vi "pco.camera_FloatingMean_Example_IMAQ.vi"() -> ()   [LabVIEW 2019]
uses:
  pco.camera/Camera.lvclass
  <vilib>/vision/NI_Vision_Development_Module.lvlib
panel:
  out "nominatorU64":u64 format="%x"
  out "denominatorU64":u64 format="%x"
  out "currentImage":T1(plugin-control)
  out "nominatorU32":u64 format="%x"
  out "denominatorU32":u64 format="%x"
  in  "averageCount":u8=10 caption="Average Count" min=2
  out "Image":T1(plugin-control)
  in  "data_format":T2(ring)=enum."Mono16"
  out "Recorded Images":u32
  in  "Quit":bool
  in  "roiY1":u64=2048 min=2 max=20000 step=1
  in  "roiX1":u64=2048 min=2 max=20000 step=1
  in  "roiY0":u64=1 min=1 max=1039 step=1
  in  "roiX0":u64=1 min=1 max=1391 step=1
  out "Image Height":u64
  out "Image Width":u64
  in  "dwImgCount":u32=10 caption="Fifo Buffer Size" max=4023
  out "Error":errorcluster {"code" format="%x"}
  # "This example shows how to compute and show a floating mean live image.\nHere the camera class is operated in fifo mode to always get next image in buffer.\nThe Average Count defines the number of images that will be averaged.\nAveraging is done by fetiching one image and using average image from previous iteration\n(avg_n = (1-1/avg_count)*avg_(n-1) + (1/avg_count)*image_n)\n\nIt is a good starting point for writing own applications.\nBut it will not be fail save, i.e. doesnt react on errors, just handles them forward to the end\n\nUsage:\nSelect your required fifo buffer size and image format and start the program.\nOnce started, the camera class will be initialized and image record will start automatically.\nInside the acquisition loop the program calculates the floating average image shows it.\nThe average count can be changed at any time.\nBy using the ROI parameters you can crop the image to select certain regions\n\nBy clicking Quit Application the record will stop and will force an exit of the camera class"
  # "pco.labview"
  # "Camera Setup"
  # "Recording Control"
  # "Parameters for image readout"
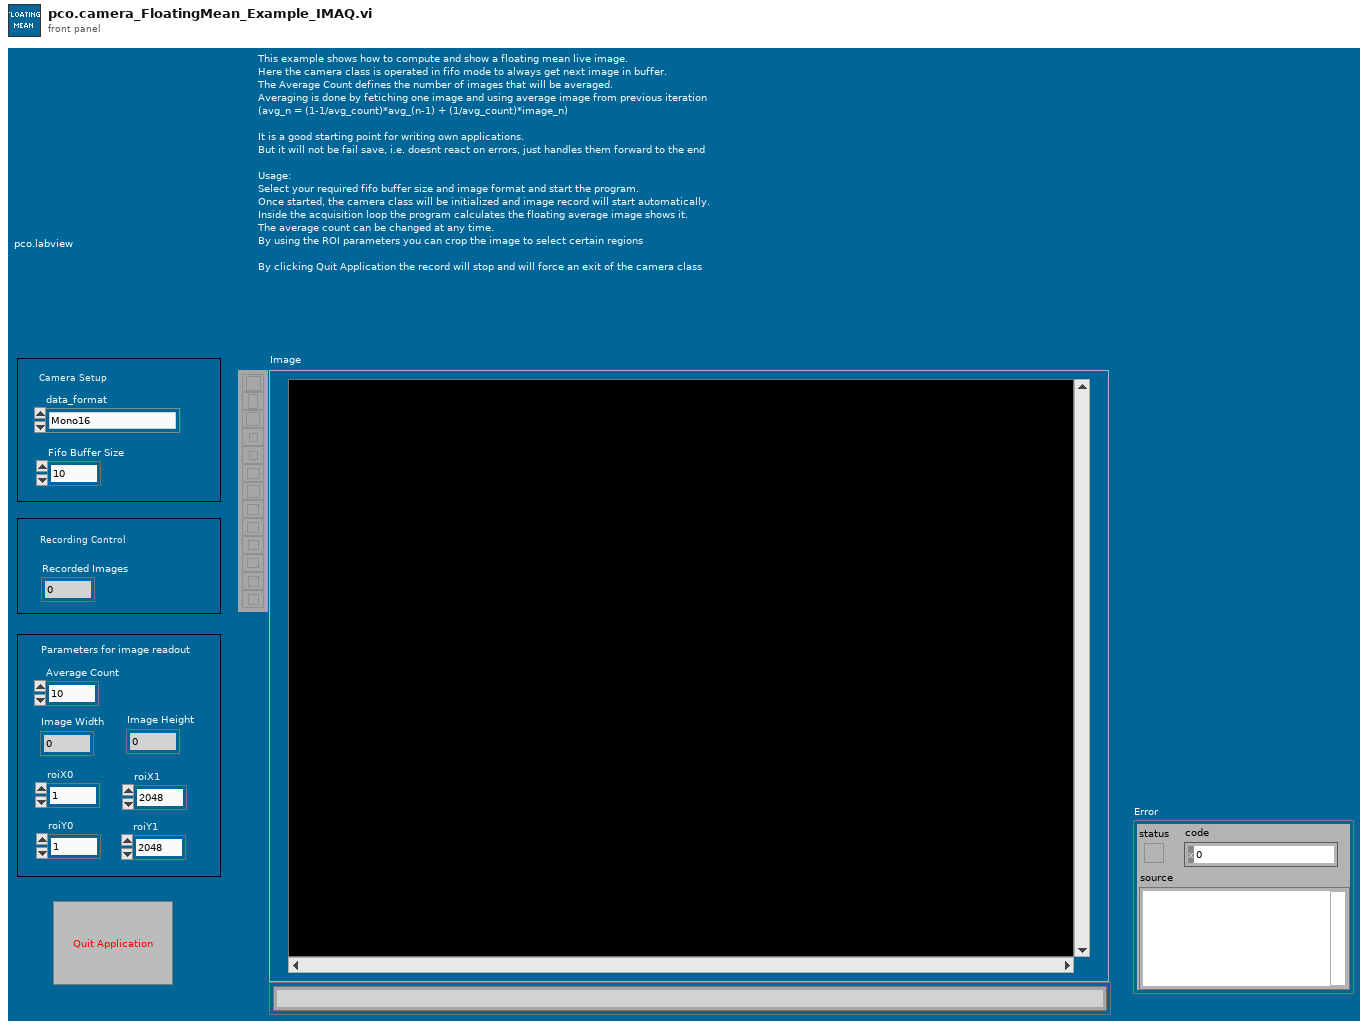
[diagram p1: front panel]
types:
  T1 = typedef "IMAQ Image.ctl" = refnum<image>
  T2 = enum16{"Undefined", "Mono8", "Mono16", "BGRA8", "RGBA8", "BGRA16", "RGBA16", "CompressedMono8"}
  T3 = enum8{"Enabled", "Disabled", "Disabled and Grayed Out"}
  T4 = enum16{"sequence", "sequence non blocking", "ring buffer", "fifo", "sequence_dpcore", "sequence_non_blocking_dpcore", "ring_buffer_dpcore", "fifo_dpcore", "tif", "multitif", "pcoraw", "b16", "dicom", "multidicom"}
  T5 = typedef "Image Type" = u32
  T6 = typedef "Camera.lvclass/binning.ctl" = cluster{"vert":u16, "horz":u16}
  T7 = cluster{"exposure_time_s":dbl, "delay_time_s":dbl, "roi":cluster{"x0":u64, "y0":u64, "x1":u64, "y1":u64}, "timestamp_mode":u16, "pixelrate":u32, "trigger_mode":u16, "acquire_mode":u16, "metadata_mode":u16, "noisefilter_mode":u16, "binning":T6}
  T8 = typedef "Color (U64)" = cluster{"Plane 3 (Blue)":u16, "Plane 2 (Green)":u16, "Plane 1 (Red)":u16, "Plane 4 (alpha)":u16}
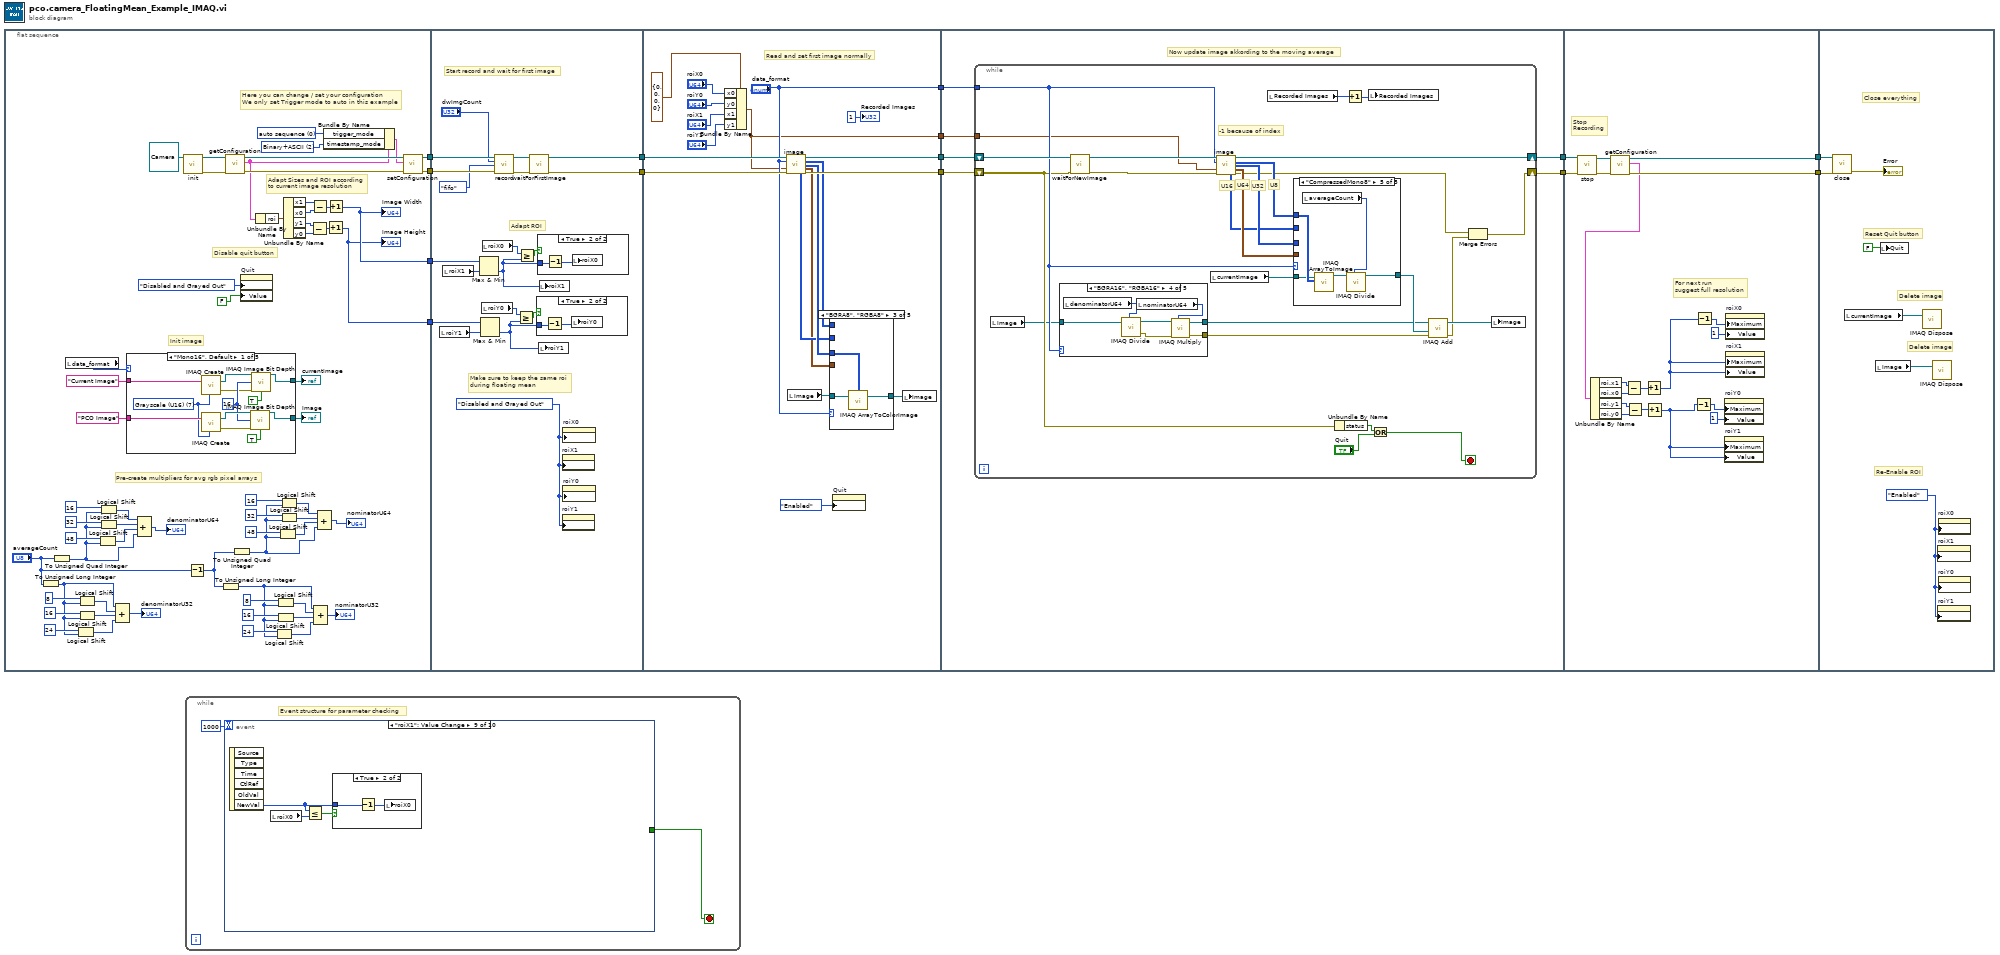
[diagram p0: block diagram]
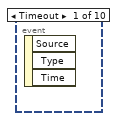
[diagram p2: hidden frame]
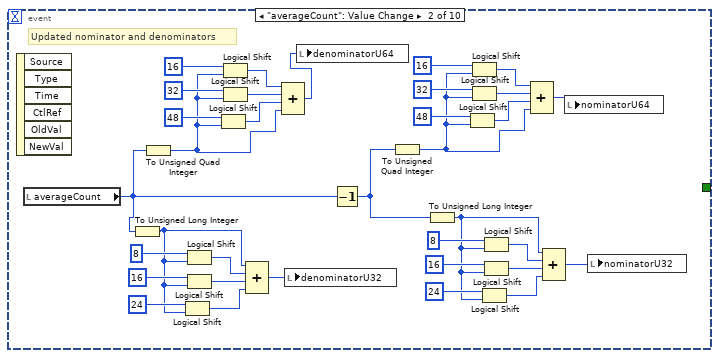
[diagram p3: hidden frame]
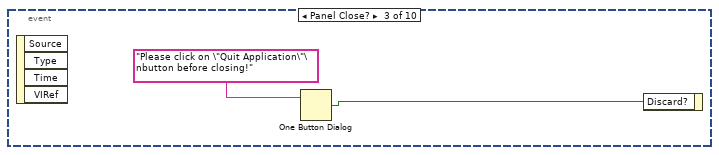
[diagram p4: hidden frame]
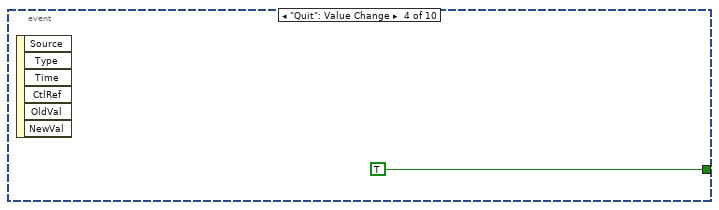
[diagram p5: hidden frame]
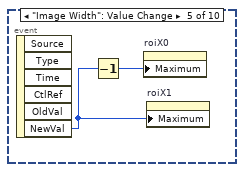
[diagram p6: hidden frame]
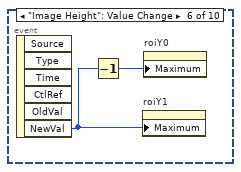
[diagram p7: hidden frame]
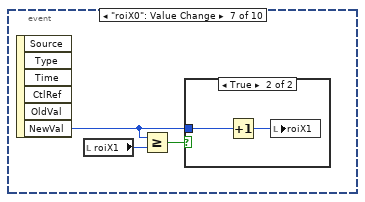
[diagram p8: hidden frame]
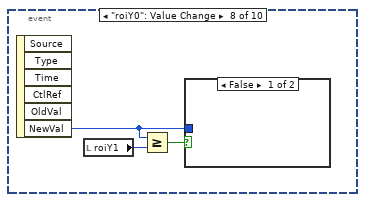
[diagram p10: hidden frame]
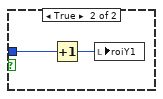
[diagram p11: hidden frame]
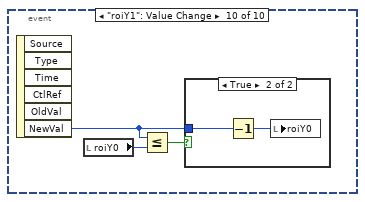
[diagram p13: hidden frame]
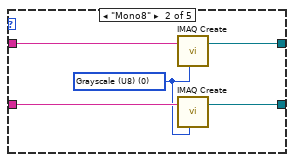
[diagram p15: hidden frame]
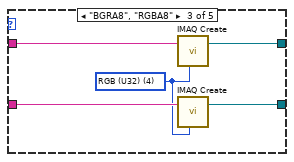
[diagram p16: hidden frame]
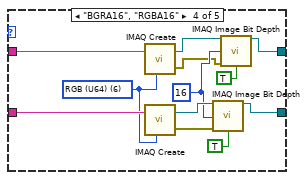
[diagram p17: hidden frame]
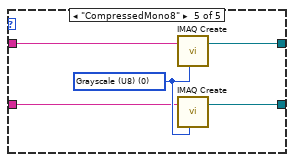
[diagram p18: hidden frame]
diagram:
  n1 = flat-sequence {
    tunnel: [w68] -> w14
    tunnel: [w67] -> w13
    tunnel: [w16] -> w2
    tunnel: [w15] -> w1
    tunnel: w14 -> [w133]
    tunnel: w13 -> [w132]
    tunnel: [w127] -> w12
    tunnel: [w126] -> w11
    tunnel: w2 -> [w123]
    tunnel: w1 -> [w121]
    tunnel: w12 -> [w155]
    tunnel: w11 -> [w154]
    tunnel: [w150] -> w10
    tunnel: [w151] -> w9
    tunnel: ["data_format"] -> w4
    tunnel: [w138] -> w3
    tunnel: w10 -> [w176]
    tunnel: w9 -> [w177]
    tunnel: [w175] -> w8
    tunnel: [w174] -> w6
    tunnel: w4 -> [w173]
    tunnel: w3 -> [w172]
    tunnel: w8 -> [w281]
    tunnel: [w276] -> w7
    tunnel: w6 -> [w280]
    tunnel: [w277] -> w5
    tunnel: w7 -> [w286]
    tunnel: w5 -> [w285]
    frame #0 {
      w58 = u16 2 items=["OFF", "Binary", "Binary+ASCII", "ASCII"] ("TimestampMode")
      w72 = u16 0 items=["auto sequence"=0, "software trigger"=1, "external exposure start & software trigger"=2, "external exposure control"=3, "external synchronized"=4, "fast external exposure control"=5, "external CDS control"=6, "slow external exposure control"=7, "external synchronized HDSDI"=258] ("TriggerMode")
      # "Pre-create multipliers for avg rgb pixel arrays"
      # "Init image"
      # "Adapt Sizes and ROI according\nto current image resolution"
      # "Disable quit button"
      # "Here you can change / set your configuration\nWe only set Trigger mode to auto in this example"
      n2 = To Unsigned Long Integer(number="averageCount") -> (unsigned 32bit integer=w38:u32)
      n3 = To Unsigned Quad Integer(1:"averageCount") -> (0:w18:u64)
      n4 = local read "data_format"() -> (w55:T2)
      n5 = Logical Shift(y=u32 24, x=w38) -> (x << y=w49:u32)
      n6 = Logical Shift(y=u32 8, x=w38) -> (x << y=w47:u32)
      n7 = Logical Shift(y=u32 16, x=w38) -> (x << y=w48:u32)
      n8 = Logical Shift(y=u32 48, x=w18) -> (x << y=w31:u64)
      n9 = Logical Shift(y=u32 16, x=w18) -> (x << y=w29:u64)
      n10 = Logical Shift(y=u32 32, x=w18) -> (x << y=w30:u64)
      n11 = Compound Arithmetic op=ADD(w38, w47, w48, w49) -> (→"denominatorU32":u32)
      n12 = case shown="\"Mono16\", Default" w55 {
        tunnel: "PCO Image" ("Image Name") -> [w87 w90 w95 w109 w112]
        tunnel: [w81 w92 w97 w103 w114] -> w54
        tunnel: [w76 w91 w96 w99 w111] -> w36
        tunnel: "Current Image" ("Image Name") -> [w85 w89 w93 w107 w110]
        frame "Mono16", Default {
          w79 = u32 16 ("Bit Depth (0)")
          w86 = T5 7 items=["Grayscale (U8)", "Grayscale (I16)", "Grayscale (SGL)", "Complex (CSG)", "RGB (U32)", "HSL (U32)", "RGB (U64)", "Grayscale (U16)"] ("Image Type")
          n13 = call "IMAQ Create"("Image Name"=w85, "Image Type"=w86) -> ("New Image"=w78:T1, "error out"=w77:errorcluster)  [unwired: 3 in]
          n14 = call "IMAQ Create"("Image Name"=w87, "Image Type"=w86) -> ("New Image"=w83:T1, "error out"=w82:errorcluster)  [unwired: 3 in]
          n15 = call "IMAQ Image Bit Depth"("Image"=w83, "Bit Depth (0)"=w79, "error in (no error)"=w82, "Get/Set Bit Depth? (Set)"=TRUE) -> ("Image Out"=w81:T1)  [unwired: 9 in, 2 out]
          n16 = call "IMAQ Image Bit Depth"("Image"=w78, "Bit Depth (0)"=w79, "error in (no error)"=w77, "Get/Set Bit Depth? (Set)"=TRUE) -> ("Image Out"=w76:T1)  [unwired: 9 in, 2 out]
        }
        frame "Mono8" {
          w88 = T5 0 items=["Grayscale (U8)", "Grayscale (I16)", "Grayscale (SGL)", "Complex (CSG)", "RGB (U32)", "HSL (U32)", "RGB (U64)", "Grayscale (U16)"] ("Image Type")
          n17 = call "IMAQ Create"("Image Name"=w89, "Image Type"=w88) -> ("New Image"=w91:T1)  [unwired: 3 in, 1 out]
          n18 = call "IMAQ Create"("Image Name"=w90, "Image Type"=w88) -> ("New Image"=w92:T1)  [unwired: 3 in, 1 out]
        }
        frame "BGRA8", "RGBA8" {
          w94 = T5 4 items=["Grayscale (U8)", "Grayscale (I16)", "Grayscale (SGL)", "Complex (CSG)", "RGB (U32)", "HSL (U32)", "RGB (U64)", "Grayscale (U16)"] ("Image Type")
          n19 = call "IMAQ Create"("Image Name"=w93, "Image Type"=w94) -> ("New Image"=w96:T1)  [unwired: 3 in, 1 out]
          n20 = call "IMAQ Create"("Image Name"=w95, "Image Type"=w94) -> ("New Image"=w97:T1)  [unwired: 3 in, 1 out]
        }
        frame "BGRA16", "RGBA16" {
          w101 = u32 16 ("Bit Depth (0)")
          w108 = T5 6 items=["Grayscale (U8)", "Grayscale (I16)", "Grayscale (SGL)", "Complex (CSG)", "RGB (U32)", "HSL (U32)", "RGB (U64)", "Grayscale (U16)"] ("Image Type")
          n21 = call "IMAQ Create"("Image Name"=w107, "Image Type"=w108) -> ("New Image"=w100:T1, "error out"=w98:errorcluster)  [unwired: 3 in]
          n22 = call "IMAQ Create"("Image Name"=w109, "Image Type"=w108) -> ("New Image"=w105:T1, "error out"=w104:errorcluster)  [unwired: 3 in]
          n23 = call "IMAQ Image Bit Depth"("Image"=w105, "Bit Depth (0)"=w101, "error in (no error)"=w104, "Get/Set Bit Depth? (Set)"=TRUE) -> ("Image Out"=w103:T1)  [unwired: 9 in, 2 out]
          n24 = call "IMAQ Image Bit Depth"("Image"=w100, "Bit Depth (0)"=w101, "error in (no error)"=w98, "Get/Set Bit Depth? (Set)"=TRUE) -> ("Image Out"=w99:T1)  [unwired: 9 in, 2 out]
        }
        frame "CompressedMono8" {
          w113 = T5 0 items=["Grayscale (U8)", "Grayscale (I16)", "Grayscale (SGL)", "Complex (CSG)", "RGB (U32)", "HSL (U32)", "RGB (U64)", "Grayscale (U16)"] ("Image Type")
          n25 = call "IMAQ Create"("Image Name"=w110, "Image Type"=w113) -> ("New Image"=w111:T1)  [unwired: 3 in, 1 out]
          n26 = call "IMAQ Create"("Image Name"=w112, "Image Type"=w113) -> ("New Image"=w114:T1)  [unwired: 3 in, 1 out]
        }
      }
      "Image" <- w54
      "currentImage" <- w36
      n27 = Compound Arithmetic op=ADD(w29, w30, w31, w18) -> (→"denominatorU64":u64)
      n28 = call-dynamic "init.vi"("Camera in"=refnum<class "Camera.lvclass"> refnum ("PCOCamera in")) -> ("Camera out"=w74:refnum<class "Camera.lvclass">, "error out"=w73:errorcluster)  [unwired: 8 in]
      n29 = Decrement(x="averageCount") -> (x-1=w19:u8)
      n30 = To Unsigned Long Integer(number=w19) -> (unsigned 32bit integer=w37:u32)
      n31 = call-dynamic "getConfiguration.vi"("error in (no error)"=w73, "Camera in"=w74) -> ("error out"=w70:errorcluster, "configuration"=w66:T7, "Camera out"=w71:refnum<class "Camera.lvclass">)  [unwired: 7 in]
      n32 = To Unsigned Quad Integer(1:w19) -> (0:w17:u64)
      n33 = property on="Quit" class="Bool (strict)"("DisabledEnum"=T3."Disabled and Grayed Out" ("Disabled"), "Value"=FALSE ("Stop")) -> ()  [unwired: 2 in, 2 out]
      n34 = Unbundle By Name(w66) -> ("roi"=w65:cluster{"x0":u64, "y0":u64, "x1":u64, "y1":u64})
      n35 = Logical Shift(y=u32 24, x=w37) -> (x << y=w42:u32)
      n36 = Logical Shift(y=u32 8, x=w37) -> (x << y=w40:u32)
      n37 = Logical Shift(y=u32 16, x=w37) -> (x << y=w41:u32)
      n38 = Logical Shift(y=u32 48, x=w17) -> (x << y=w23:u64)
      n39 = Logical Shift(y=u32 16, x=w17) -> (x << y=w25:u64)
      n40 = Logical Shift(y=u32 32, x=w17) -> (x << y=w24:u64)
      n41 = Unbundle By Name(w65) -> ("x1"=w63:u64, "x0"=w64:u64, "y1"=w61:u64, "y0"=w62:u64)
      n42 = Subtract(x=w61, y=w62) -> (x-y=w59:u64)
      n43 = Subtract(x=w63, y=w64) -> (x-y=w60:u64)
      n44 = Compound Arithmetic op=ADD(w37, w40, w41, w42) -> (→"nominatorU32":u32)
      n45 = Compound Arithmetic op=ADD(w25, w24, w23, w17) -> (→"nominatorU64":u64)
      n46 = Bundle By Name(cluster=w66, "trigger_mode"=w72, "timestamp_mode"=w58) -> (w69:T7)
      n47 = Increment(x=w59) -> (x+1=w15:u64)
      "Image Height" <- w15
      n48 = Increment(x=w60) -> (x+1=w16:u64)
      "Image Width" <- w16
      n49 = call-dynamic "setConfiguration.vi"("error in (no error)"=w70, "configuration"=w69, "Camera in"=w71) -> ("error out"=w67:errorcluster, "Camera out"=w68:refnum<class "Camera.lvclass">)  [unwired: 7 in]
    }
    frame #1 {
      w125 = T3."Disabled and Grayed Out" ("Disabled")
      # "Adapt ROI"
      # "Make sure to keep the same roi\nduring floating mean"
      # "Start record and wait for first image"
      n50 = local read "roiY1"() -> (w122:u64)
      n51 = local read "roiX1"() -> (w124:u64)
      n52 = Max & Min(x=w123, y=w124) -> (min(x,y)=w118:u64)  [unwired: 1 out]
      n53 = Max & Min(x=w121, y=w122) -> (min(x,y)=w115:u64)  [unwired: 1 out]
      n54 = local read "roiY0"() -> (w116:u64)
      n55 = local read "roiX0"() -> (w120:u64)
      n56 = call-dynamic "record.vi"("Camera in"=w133, "num_images"="dwImgCount", "record_mode"=T4."fifo", "error in (no error)"=w132) -> ("Camera out"=w128:refnum<class "Camera.lvclass">, "error out"=w129:errorcluster)  [unwired: 10 in]
      n57 = Greater Or Equal?(x=w116, y=w115) -> (x >= y?=w117:bool)
      n58 = Greater Or Equal?(x=w120, y=w118) -> (x >= y?=w119:bool)
      n59 = call-dynamic "waitForFirstImage.vi"("error in (no error)"=w129, "Camera in"=w128) -> ("error out"=w126:errorcluster, "Camera out"=w127:refnum<class "Camera.lvclass">)  [unwired: 8 in]
      n60 = case shown="True" w117 {
        tunnel: w115 -> [_ w135]
        frame False {
        }
        frame True {
          n61 = Decrement(x=w135) -> (x-1=w134:u64)
          n62 = local write "roiY0"(w134) -> ()
        }
      }
      n63 = case shown="True" w119 {
        tunnel: w118 -> [_ w137]
        frame False {
        }
        frame True {
          n64 = Decrement(x=w137) -> (x-1=w136:u64)
          n65 = local write "roiX0"(w136) -> ()
        }
      }
      n66 = local write "roiY1"(w115) -> ()
      n67 = local write "roiX1"(w118) -> ()
      n68 = property on="roiX1" class="DigNum (strict)"("DisabledEnum"=w125) -> ()  [unwired: 2 in, 2 out]
      n69 = property on="roiY1" class="DigNum (strict)"("DisabledEnum"=w125) -> ()  [unwired: 2 in, 2 out]
      n70 = property on="roiX0" class="DigNum (strict)"("DisabledEnum"=w125) -> ()  [unwired: 2 in, 2 out]
      n71 = property on="roiY0" class="DigNum (strict)"("DisabledEnum"=w125) -> ()  [unwired: 2 in, 2 out]
    }
    frame #2 {
      # "Read and set first image normally"
      n72 = Bundle By Name(cluster=cluster{"x0":u64, "y0":u64, "x1":u64, "y1":u64} {"x0"=0, "y0"=0, "x1"=0, "y1"=0} ("roi"), "x0"="roiX0", "y0"="roiY0", "x1"="roiX1", "y1"="roiY1") -> (w138:cluster{"x0":u64, "y0":u64, "x1":u64, "y1":u64})
      n73 = call-dynamic "image.vi"("Camera in"=w155, "data_format"="data_format", "roi"=w138, "error in (no error)"=w154) -> ("Camera out"=w150:refnum<class "Camera.lvclass">, "image (U8)"=w148:u8[][], "image (U32)"=w147:u32[][], "image (U64)"=w145:T8[][], "raw_image (U16)"=w146:u16[][], "error out"=w151:errorcluster)  [unwired: 4 in, 2 out]
      n74 = local read "Image"() -> (w153:T1)
      n75 = case shown="\"BGRA8\", \"RGBA8\"" "data_format" {
        tunnel: w153 -> [w159 w162 w163 w168 w171]
        tunnel: [w157 w160 w165 w166 w170] -> w144
        tunnel: w145 -> [_ _ _ w167 _]
        tunnel: w147 -> [_ _ w164 _ _]
        tunnel: w148 -> [_ w161 _ _ w169]
        tunnel: w146 -> [w158 _ _ _ _]
        frame "Mono16", Default {
          n76 = call "IMAQ ArrayToImage"("Image Pixels (U16)"=w158, "Image"=w159) -> ("Image Out"=w157:T1)  [unwired: 8 in, 1 out]
        }
        frame "Mono8" {
          n77 = call "IMAQ ArrayToImage"("Image Pixels (U8)"=w161, "Image"=w162) -> ("Image Out"=w160:T1)  [unwired: 8 in, 1 out]
        }
        frame "BGRA8", "RGBA8" {
          n78 = call "IMAQ ArrayToColorImage"("Image Pixels (U32)"=w164, "Image"=w163) -> ("Image Out"=w165:T1)  [unwired: 3 in, 1 out]
        }
        frame "BGRA16", "RGBA16" {
          n79 = call "IMAQ ArrayToColorImage"("Image"=w168, "Image Pixels (U64)"=w167) -> ("Image Out"=w166:T1)  [unwired: 3 in, 1 out]
        }
        frame "CompressedMono8" {
          n80 = call "IMAQ ArrayToImage"("Image Pixels (U8)"=w169, "Image"=w171) -> ("Image Out"=w170:T1)  [unwired: 8 in, 1 out]
        }
      }
      n81 = property on="Quit" class="Bool (strict)"("DisabledEnum"=T3."Enabled" ("Disabled")) -> ()  [unwired: 2 in, 2 out]
      n82 = local write "Image"(w144) -> ()
      "Recorded Images" <- u32 1 ("Recorded Images")
    }
    frame #3 {
      # "Now update image akkording to the moving average"
      n83 = while {
        shift-right: [w202] -> w175
        shift-left: w176 -> [w201]
        shift-right: [w182] -> w174
        shift-left: w177 -> [w188]
        tunnel: w173 -> [w191]
        tunnel: w172 -> [w178]
        stop <- w185 stop-if-true
        # "-1 because of index"
        # "U64"
        # "U32"
        # "U16"
        # "U8"
        n84 = local read "Image"() -> (w181:T1)
        n85 = case shown="\"BGRA16\", \"RGBA16\"" w191 {
          tunnel: w181 -> [w206 w214 w222 w229 w235]
          tunnel: [w205 w212 w219 w228 w233] -> w179
          tunnel: [w203 w210 w217 w226 w231] -> w189
          frame "Mono16", Default {
            n86 = local read "averageCount"() -> (w208:u8)
            n87 = call "IMAQ Divide"("Image Src A"=w206, "Constant"=w208) -> ("Image Dst Out"=w209:T1, "error out"=w204:errorcluster)  [unwired: 5 in]
            n88 = Decrement(x=w208) -> (x-1=w207:u8)
            n89 = call "IMAQ Multiply"("Image Src A"=w209, "Constant"=w207, "error in (no error)"=w204) -> ("Image Dst Out"=w205:T1, "error out"=w203:errorcluster)  [unwired: 4 in]
          }
          frame "Mono8" {
            n90 = local read "averageCount"() -> (w213:u8)
            n91 = call "IMAQ Divide"("Image Src A"=w214, "Constant"=w213) -> ("Image Dst Out"=w216:T1, "error out"=w211:errorcluster)  [unwired: 5 in]
            n92 = Decrement(x=w213) -> (x-1=w215:u8)
            n93 = call "IMAQ Multiply"("Image Src A"=w216, "Constant"=w215, "error in (no error)"=w211) -> ("Image Dst Out"=w212:T1, "error out"=w210:errorcluster)  [unwired: 4 in]
          }
          frame "BGRA8", "RGBA8" {
            n94 = local read "denominatorU32"() -> (w221:u64)
            n95 = call "IMAQ Divide"("Image Src A"=w222, "Constant"=w221) -> ("Image Dst Out"=w223:T1, "error out"=w218:errorcluster)  [unwired: 5 in]
            n96 = local read "nominatorU32"() -> (w220:u64)
            n97 = call "IMAQ Multiply"("Image Src A"=w223, "Constant"=w220, "error in (no error)"=w218) -> ("Image Dst Out"=w219:T1, "error out"=w217:errorcluster)  [unwired: 4 in]
          }
          frame "BGRA16", "RGBA16" {
            n98 = local read "denominatorU64"() -> (w225:u64)
            n99 = call "IMAQ Divide"("Image Src A"=w229, "Constant"=w225) -> ("Image Dst Out"=w230:T1, "error out"=w227:errorcluster)  [unwired: 5 in]
            n100 = local read "nominatorU64"() -> (w224:u64)
            n101 = call "IMAQ Multiply"("Image Src A"=w230, "Constant"=w224, "error in (no error)"=w227) -> ("Image Dst Out"=w228:T1, "error out"=w226:errorcluster)  [unwired: 4 in]
          }
          frame "CompressedMono8" {
            n102 = local read "averageCount"() -> (w234:u8)
            n103 = call "IMAQ Divide"("Image Src A"=w235, "Constant"=w234) -> ("Image Dst Out"=w237:T1, "error out"=w232:errorcluster)  [unwired: 5 in]
            n104 = Decrement(x=w234) -> (x-1=w236:u8)
            n105 = call "IMAQ Multiply"("Image Src A"=w237, "Constant"=w236, "error in (no error)"=w232) -> ("Image Dst Out"=w233:T1, "error out"=w231:errorcluster)  [unwired: 4 in]
          }
        }
        n106 = call-dynamic "waitForNewImage.vi"("error in (no error)"=w188, "Camera in"=w201) -> ("error out"=w197:errorcluster, "Camera out"=w198:refnum<class "Camera.lvclass">)  [unwired: 8 in]
        n107 = local read "currentImage"() -> (w190:T1)
        n108 = call-dynamic "image.vi"("Camera in"=w198, "data_format"=w191, "roi"=w178, "error in (no error)"=w197) -> ("Camera out"=w202:refnum<class "Camera.lvclass">, "image (U8)"=w196:u8[][], "image (U32)"=w194:u32[][], "image (U64)"=w195:T8[][], "raw_image (U16)"=w193:u16[][], "error out"=w183:errorcluster)  [unwired: 4 in, 2 out]
        n109 = local read "Recorded Images"() -> (w200:u32)
        n110 = case shown="\"CompressedMono8\"" w191 {
          tunnel: [w239 w245 w250 w255 w259] -> w180
          tunnel: w195 -> [_ _ _ w257 _]
          tunnel: w194 -> [_ _ w252 _ _]
          tunnel: w196 -> [_ w247 _ _ w262]
          tunnel: w193 -> [w242 _ _ _ _]
          tunnel: w190 -> [w238 w243 w248 w253 w258]
          frame "Mono16", Default {
            n111 = local read "averageCount"() -> (w240:u8)
            n112 = call "IMAQ ArrayToImage"("Image Pixels (U16)"=w242, "Image"=w238) -> ("Image Out"=w241:T1)  [unwired: 8 in, 1 out]
            n113 = call "IMAQ Divide"("Image Src A"=w241, "Constant"=w240) -> ("Image Dst Out"=w239:T1)  [unwired: 5 in, 1 out]
          }
          frame "Mono8" {
            n114 = local read "averageCount"() -> (w244:u8)
            n115 = call "IMAQ ArrayToImage"("Image Pixels (U8)"=w247, "Image"=w243) -> ("Image Out"=w246:T1)  [unwired: 8 in, 1 out]
            n116 = call "IMAQ Divide"("Image Src A"=w246, "Constant"=w244) -> ("Image Dst Out"=w245:T1)  [unwired: 5 in, 1 out]
          }
          frame "BGRA8", "RGBA8" {
            n117 = local read "denominatorU32"() -> (w249:u64)
            n118 = call "IMAQ ArrayToColorImage"("Image Pixels (U32)"=w252, "Image"=w248) -> ("Image Out"=w251:T1)  [unwired: 3 in, 1 out]
            n119 = call "IMAQ Divide"("Image Src A"=w251, "Constant"=w249) -> ("Image Dst Out"=w250:T1)  [unwired: 5 in, 1 out]
          }
          frame "BGRA16", "RGBA16" {
            n120 = local read "denominatorU64"() -> (w254:u64)
            n121 = call "IMAQ ArrayToColorImage"("Image"=w253, "Image Pixels (U64)"=w257) -> ("Image Out"=w256:T1)  [unwired: 3 in, 1 out]
            n122 = call "IMAQ Divide"("Image Src A"=w256, "Constant"=w254) -> ("Image Dst Out"=w255:T1)  [unwired: 5 in, 1 out]
          }
          frame "CompressedMono8" {
            n123 = local read "averageCount"() -> (w260:u8)
            n124 = call "IMAQ ArrayToImage"("Image Pixels (U8)"=w262, "Image"=w258) -> ("Image Out"=w261:T1)  [unwired: 8 in, 1 out]
            n125 = call "IMAQ Divide"("Image Src A"=w261, "Constant"=w260) -> ("Image Dst Out"=w259:T1)  [unwired: 5 in, 1 out]
          }
        }
        n126 = Unbundle By Name(w188) -> ("status"=w187:bool)
        n127 = Increment(x=w200) -> (x+1=w199:u32)
        n128 = local write "Recorded Images"(w199) -> ()
        n129 = Or(x=w187, y="Quit") -> (x .or. y?=w185:bool)
        n130 = call "IMAQ Add"("Image Src A"=w179, "Image Src B"=w180, "error in (no error)"=w189) -> ("Image Dst Out"=w192:T1, "error out"=w184:errorcluster)  [unwired: 4 in]
        n131 = Merge Errors(w183, w184) -> (w182:errorcluster)
        n132 = local write "Image"(w192) -> ()
      }
    }
    frame #4 {
      # "For next run \nsuggest full resolution"
      # "Stop \nRecording"
      n133 = call-dynamic "stop.vi"("error in (no error)"=w280, "Camera in"=w281) -> ("error out"=w278:errorcluster, "Camera out"=w279:refnum<class "Camera.lvclass">)  [unwired: 8 in]
      n134 = call-dynamic "getConfiguration.vi"("error in (no error)"=w278, "Camera in"=w279) -> ("error out"=w277:errorcluster, "configuration"=w263:T7, "Camera out"=w276:refnum<class "Camera.lvclass">)  [unwired: 7 in]
      n135 = Unbundle By Name(w263) -> ("roi.x1"=w269:u64, "roi.x0"=w268:u64, "roi.y1"=w267:u64, "roi.y0"=w266:u64)
      n136 = Subtract(x=w269, y=w268) -> (x-y=w270:u64)
      n137 = Subtract(x=w267, y=w266) -> (x-y=w271:u64)
      n138 = Increment(x=w270) -> (x+1=w274:u64)
      n139 = Increment(x=w271) -> (x+1=w273:u64)
      n140 = Decrement(x=w273) -> (x-1=w272:u64)
      n141 = Decrement(x=w274) -> (x-1=w275:u64)
      n142 = property on="roiY0" class="DigNum (strict)"("Maximum"=w272, "Value"=u64 1 ("roiY0")) -> ()  [unwired: 2 in, 2 out]
      n143 = property on="roiY1" class="DigNum (strict)"("Maximum"=w273, "Value"=w273) -> ()  [unwired: 2 in, 2 out]
      n144 = property on="roiX0" class="DigNum (strict)"("Maximum"=w275, "Value"=u64 1 ("roiX0")) -> ()  [unwired: 2 in, 2 out]
      n145 = property on="roiX1" class="DigNum (strict)"("Maximum"=w274, "Value"=w274) -> ()  [unwired: 2 in, 2 out]
    }
    frame #5 {
      w282 = T3."Enabled" ("Disabled")
      # "Re-Enable ROI"
      # "Delete image"
      # "Delete image"
      # "Reset Quit button"
      # "Close everything"
      n146 = call-dynamic "close.vi"("error in (no error)"=w285, "Camera in"=w286) -> ("error out"=→"Error":errorcluster)  [unwired: 9 in]
      n147 = local read "currentImage"() -> (w283:T1)
      n148 = local read "Image"() -> (w284:T1)
      n149 = local write "Quit"(FALSE ("Stop")) -> ()
      n150 = call "IMAQ Dispose"("Image"=w283) -> ()  [unwired: 5 in, 1 out]
      n151 = call "IMAQ Dispose"("Image"=w284) -> ()  [unwired: 5 in, 1 out]
      n152 = property on="roiX1" class="DigNum (strict)"("DisabledEnum"=w282) -> ()  [unwired: 2 in, 2 out]
      n153 = property on="roiY1" class="DigNum (strict)"("DisabledEnum"=w282) -> ()  [unwired: 2 in, 2 out]
      n154 = property on="roiX0" class="DigNum (strict)"("DisabledEnum"=w282) -> ()  [unwired: 2 in, 2 out]
      n155 = property on="roiY0" class="DigNum (strict)"("DisabledEnum"=w282) -> ()  [unwired: 2 in, 2 out]
    }
  }
  n156 = while {
    stop <- w289 stop-if-true
    # "Event structure for parameter checking"
    n157 = event shown="[8] \"roiX1\": Value Change" {
      selector: _ -> [_ _ _ _ _ _ _ _ _ _]
      dyn-events: _ -> [_ _ _ _ _ _ _ _ _ _]
      timeout: 1000 -> [_ _ _ _ _ _ _ _ _ _]
      tunnel: [_ _ _ TRUE _ _ _ _ _ _] -> w289
      event Timeout {
        n158 = event-data() -> ()  [unwired: 1 in, 3 out]
      }
      event "averageCount": Value Change {
        # "Updated nominator and denominators"
        n159 = event-data() -> ()  [unwired: 1 in, 6 out]
        n160 = local read "averageCount"() -> (w297:u8)
        n161 = To Unsigned Long Integer(number=w297) -> (unsigned 32bit integer=w310:u32)
        n162 = To Unsigned Quad Integer(1:w297) -> (0:w294:u64)
        n163 = Logical Shift(y=u32 24, x=w310) -> (x << y=w321:u32)
        n164 = Logical Shift(y=u32 8, x=w310) -> (x << y=w319:u32)
        n165 = Logical Shift(y=u32 16, x=w310) -> (x << y=w320:u32)
        n166 = Logical Shift(y=u32 48, x=w294) -> (x << y=w300:u64)
        n167 = Logical Shift(y=u32 16, x=w294) -> (x << y=w302:u64)
        n168 = Logical Shift(y=u32 32, x=w294) -> (x << y=w301:u64)
        n169 = Compound Arithmetic op=ADD(w310, w319, w320, w321) -> (w312:u32)
        n170 = Compound Arithmetic op=ADD(w302, w301, w300, w294) -> (w295:u64)
        n171 = local write "denominatorU32"(w312) -> ()
        n172 = local write "denominatorU64"(w295) -> ()
        n173 = Decrement(x=w297) -> (x-1=w303:u8)
        n174 = To Unsigned Quad Integer(1:w303) -> (0:w293:u64)
        n175 = To Unsigned Long Integer(number=w303) -> (unsigned 32bit integer=w309:u32)
        n176 = Logical Shift(y=u32 48, x=w293) -> (x << y=w306:u64)
        n177 = Logical Shift(y=u32 16, x=w293) -> (x << y=w308:u64)
        n178 = Logical Shift(y=u32 32, x=w293) -> (x << y=w307:u64)
        n179 = Logical Shift(y=u32 24, x=w309) -> (x << y=w315:u32)
        n180 = Logical Shift(y=u32 8, x=w309) -> (x << y=w313:u32)
        n181 = Logical Shift(y=u32 16, x=w309) -> (x << y=w314:u32)
        n182 = Compound Arithmetic op=ADD(w308, w307, w306, w293) -> (w296:u64)
        n183 = Compound Arithmetic op=ADD(w309, w313, w314, w315) -> (w311:u32)
        n184 = local write "nominatorU64"(w296) -> ()
        n185 = local write "nominatorU32"(w311) -> ()
      }
      event Panel Close? {
        n186 = event-data() -> ()  [unwired: 1 in, 4 out]
        n187 = One Button Dialog(message="Please click on \"Quit Application\"\nbutton before closing!") -> (true=w325:bool)  [unwired: 1 in]
        n188 = event-data("Discard?"=w325) -> ()  [unwired: 1 in, 1 out]
      }
      event "Quit": Value Change {
        n189 = event-data() -> ()  [unwired: 1 in, 6 out]
      }
      event "Image Width": Value Change {
        n190 = event-data() -> ("NewVal"=w328:u64)  [unwired: 1 in, 5 out]
        n191 = Decrement(x=w328) -> (x-1=w329:u64)
        n192 = property on="roiX0" class="DigNum (strict)"("Maximum"=w329) -> ()  [unwired: 2 in, 2 out]
        n193 = property on="roiX1" class="DigNum (strict)"("Maximum"=w328) -> ()  [unwired: 2 in, 2 out]
      }
      event "Image Height": Value Change {
        n194 = event-data() -> ("NewVal"=w330:u64)  [unwired: 1 in, 5 out]
        n195 = Decrement(x=w330) -> (x-1=w331:u64)
        n196 = property on="roiY1" class="DigNum (strict)"("Maximum"=w330) -> ()  [unwired: 2 in, 2 out]
        n197 = property on="roiY0" class="DigNum (strict)"("Maximum"=w331) -> ()  [unwired: 2 in, 2 out]
      }
      event "roiX0": Value Change {
        n198 = event-data() -> ("NewVal"=w332:u64)  [unwired: 1 in, 5 out]
        n199 = local read "roiX1"() -> (w334:u64)
        n200 = Greater Or Equal?(x=w332, y=w334) -> (x >= y?=w333:bool)
        n201 = case shown="True" w333 {
          tunnel: w332 -> [_ w336]
          frame False {
          }
          frame True {
            n202 = Increment(x=w336) -> (x+1=w335:u64)
            n203 = local write "roiX1"(w335) -> ()
          }
        }
      }
      event "roiY0": Value Change {
        n204 = event-data() -> ("NewVal"=w337:u64)  [unwired: 1 in, 5 out]
        n205 = local read "roiY1"() -> (w339:u64)
        n206 = Greater Or Equal?(x=w337, y=w339) -> (x >= y?=w338:bool)
        n207 = case shown="False" w338 {
          tunnel: w337 -> [_ w341]
          frame False {
          }
          frame True {
            n208 = Increment(x=w341) -> (x+1=w340:u64)
            n209 = local write "roiY1"(w340) -> ()
          }
        }
      }
      event "roiX1": Value Change {
        n210 = event-data() -> ("NewVal"=w342:u64)  [unwired: 1 in, 5 out]
        n211 = local read "roiX0"() -> (w344:u64)
        n212 = Less Or Equal?(x=w342, y=w344) -> (x <= y?=w343:bool)
        n213 = case shown="True" w343 {
          tunnel: w342 -> [_ w346]
          frame False {
          }
          frame True {
            n214 = Decrement(x=w346) -> (x-1=w345:u64)
            n215 = local write "roiX0"(w345) -> ()
          }
        }
      }
      event "roiY1": Value Change {
        n216 = event-data() -> ("NewVal"=w347:u64)  [unwired: 1 in, 5 out]
        n217 = local read "roiY0"() -> (w349:u64)
        n218 = Less Or Equal?(x=w347, y=w349) -> (x <= y?=w348:bool)
        n219 = case shown="True" w348 {
          tunnel: w347 -> [_ w351]
          frame False {
          }
          frame True {
            n220 = Decrement(x=w351) -> (x-1=w350:u64)
            n221 = local write "roiY0"(w350) -> ()
          }
        }
      }
    }
  }
